vi "Single Tone Microphone Measurements (N Ch).vi"(6 "units settings":T2, 8 "error in":errorcluster, 10 "measurement settings":T4={"Band start"=20.0, "Band stop"=20000.0, "Frequency"=1000.0}, 11 "waveforms":waveform(dbl)[](array[waveform])) -> (0 "error out":errorcluster, 1 "spectra":cluster{"x0":dbl, "dx":dbl, "magnitude":dbl[]}[](array[cluster]), 2 "waveforms":waveform(dbl)[](array[waveform]), 3 "measurements":T1[](array[typedef]))   [LabVIEW 2022 SP3]
uses:
  controls/single tone microphone measurement settings.ctl
  controls/units settings - mic.ctl
  controls/measurement units.ctl
  controls/single tone microphone measurements.ctl
  <vilib>/addons/_NISVFA/_Shared subVIs/Common/SVL Set dB Reference (N Ch - 1 Ref).vi
  <vilib>/addons/_NISVFA/_Spectrum Processing/SVFA Unit Conversion (Complex) (1 Ch).vi
  <vilib>/addons/_NISVFA/_Shared subVIs/Common/SVL Set dB Reference (1 Ch).vi
  <vilib>/addons/_NISVFA/_Shared subVIs/Common/svc_Log View for Spectrum (1Ch).vi
  <vilib>/addons/_NISVFA/_Spectrum Processing/SVFA Unit Conversion (1 Ch).vi
  <vilib>/addons/_NISVFA/_Shared subVIs/Common/svc_Complex Datatype Defaults.vi
  <vilib>/addons/_NISVFA/_Shared subVIs/Common/SVL Set dB Reference (variant).vi
  <vilib>/addons/_NISVFA/_Shared subVIs/Common/svc_Unwrap Phase.vi
  <vilib>/addons/_NISVFA/_Shared subVIs/Common/svc_Convert Spectrum Array to dB.vi
  <vilib>/addons/_NISVFA/_Shared subVIs/Common/svc_Spectrum Units.vi
  <vilib>/addons/_NISVFA/_Spectrum Processing/subVIs/svfa_Conversion Utility (spectrum info).vi
  <vilib>/addons/_NISVFA/_Shared subVIs/Common/svc_Format Value (DBL).vi
  <vilib>/addons/_NISVFA/_Shared subVIs/Common/svc_Get Weighting Enum and Labels.vi
  <vilib>/addons/_NISVFA/_Shared subVIs/Common/svc_Engineering Units to Unit Label.vi
  <vilib>/addons/_NISVFA/_Shared subVIs/Common/svc_Surround NonAlpha String with Parentheses.vi
  <vilib>/dlg_ctls.llb/Space Constant.vi
  <vilib>/addons/_NISVFA/_Spectrum Processing/subVIs/svfa_Peak to RMS to Peak2Peak.vi
  <vilib>/addons/_NISVFA/_Spectrum Processing/subVIs/svfa_Mag to Mag2.vi
  <vilib>/addons/_NISVFA/_Spectrum Processing/subVIs/svfa_Linear to dB.vi
  <vilib>/addons/_NISVFA/_Spectrum Processing/subVIs/svfa_dBrefA to dBrefB.vi
  <vilib>/addons/_NISVFA/_Spectrum Processing/subVIs/svfa_Spectrum to Spectral Density.vi
  <vilib>/addons/_NISVFA/_Shared subVIs/Common/svc_Unit Label Lexical Class.vi
  <vilib>/addons/_NISVFA/_Shared subVIs/Common/svc_Window Parameters.vi
  <vilib>/addons/_NISVFA/_Shared subVIs/Common/svc_Caller VI Returned in Error Source.vi
  <vilib>/addons/Sound and Vibration/svt_Level/SVL Leq Sound Level (1 Ch).vi
  <vilib>/addons/Sound and Vibration/svt_Distortion/SVT SNR without Harmonics (Time) (1 Ch).vi
  <vilib>/addons/_NISVFA/_Spectrum Processing/SVFA Extract Single Tone Information (Complex) (1 Ch).vi
  <vilib>/Analysis/4window.llb/window parameters.vi
  <vilib>/Analysis/4window.llb/Window Properties.vi
  <vilib>/Analysis/4window.llb/Window Properties by Name.vi
  <vilib>/addons/Sound and Vibration/svt_Distortion/SoundVib_Distortion.lvlib
  <vilib>/addons/Sound and Vibration/svt_Level/SoundVib_SoundLevel.lvlib
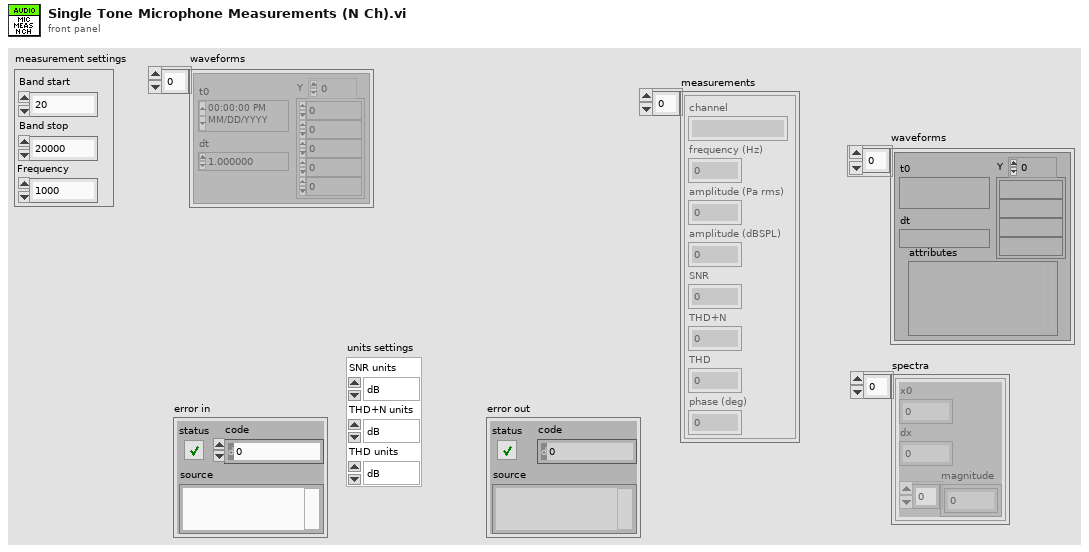
[diagram p1: front panel]
types:
  T1 = typedef "single tone microphone measurements.ctl" = cluster{"channel":string, "frequency (Hz)":dbl, "amplitude (Pa rms)":dbl, "amplitude (dBSPL)":dbl, "SNR":dbl, "THD+N":dbl, "THD":dbl, "phase (deg)":dbl}
  T2 = typedef "units settings - mic.ctl" = cluster{"SNR units":T3, "THD+N units":T3, "THD units":T3}
  T3 = typedef "measurement units.ctl" = enum32{"dB", "x/y"}
  T4 = typedef "single tone microphone measurement settings.ctl" = cluster{"Band start":dbl, "Band stop":dbl, "Frequency":dbl}
  T5 = cluster{"start frequency":dbl, "stop frequency":dbl}
  T6 = cluster{"SNR units":enum16{"dB", "linear ratio", "%"}, "detected fundamental amplitude units":enum16{"EU rms", "EU peak", "EU peak-peak"}}
  T7 = enum16{"no change", "spectrum", "spectral density"}
  T8 = cluster{"linear/dB":enum16{"no change", "linear", "dB"}, "dB reference (0: no change)":dbl, "power/magnitude":enum16{"no change", "power", "magnitude"}, "view":enum16{"no change", "rms", "peak", "peak-peak"}}
  T9 = typedef "svc_Spectrum Info.ctl" = cluster{"channel name":string, "description":string, "x-axis units":T10, "spectral info":cluster{"spectrum type":T11, "linear/dB":enum16{"linear", "dB"}, "window":u16, "window size":i32, "FFT size":i32}, "engineering units":T12, "custom label":string, "dB reference [EU]":dbl, "peak units":enum16{"rms", "peak", "peak-peak"}, "weighting filter":T13, "spectral density?":bool, "unit label":string, "spectrum skewed?":bool, "complimentary spectrum units":T14}
  T10 = typedef "svc_X-Axis Units.ctl" = u16
  T11 = typedef "svc_Spectrum Type.ctl" = enum16{"FFT Spectrum [complex]", "Amplitude [Magnitude]", "Power [Magnitude^2]", "Cross Spectrum [complex]", "Frequency Response [Complex]"}
  T12 = typedef "svc_Engineering Units Text Ring.ctl" = u16
  T13 = typedef "svc_Weighting Filter Text Ring.ctl" = u16
  T14 = typedef "svc_Complimentary Spectrum Units.ctl" = enum16{"none", "radians", "degrees", "cycles", "imaginary"}
  T15 = cluster{"complex spectrum response":cluster{"f0":dbl, "df":dbl, "complex spectrum":cdb[]}, "spectrum info":T9}
  T16 = cluster{"frequency [Hz]":dbl, "amplitude [EU pk]":dbl, "phase (deg)":dbl}
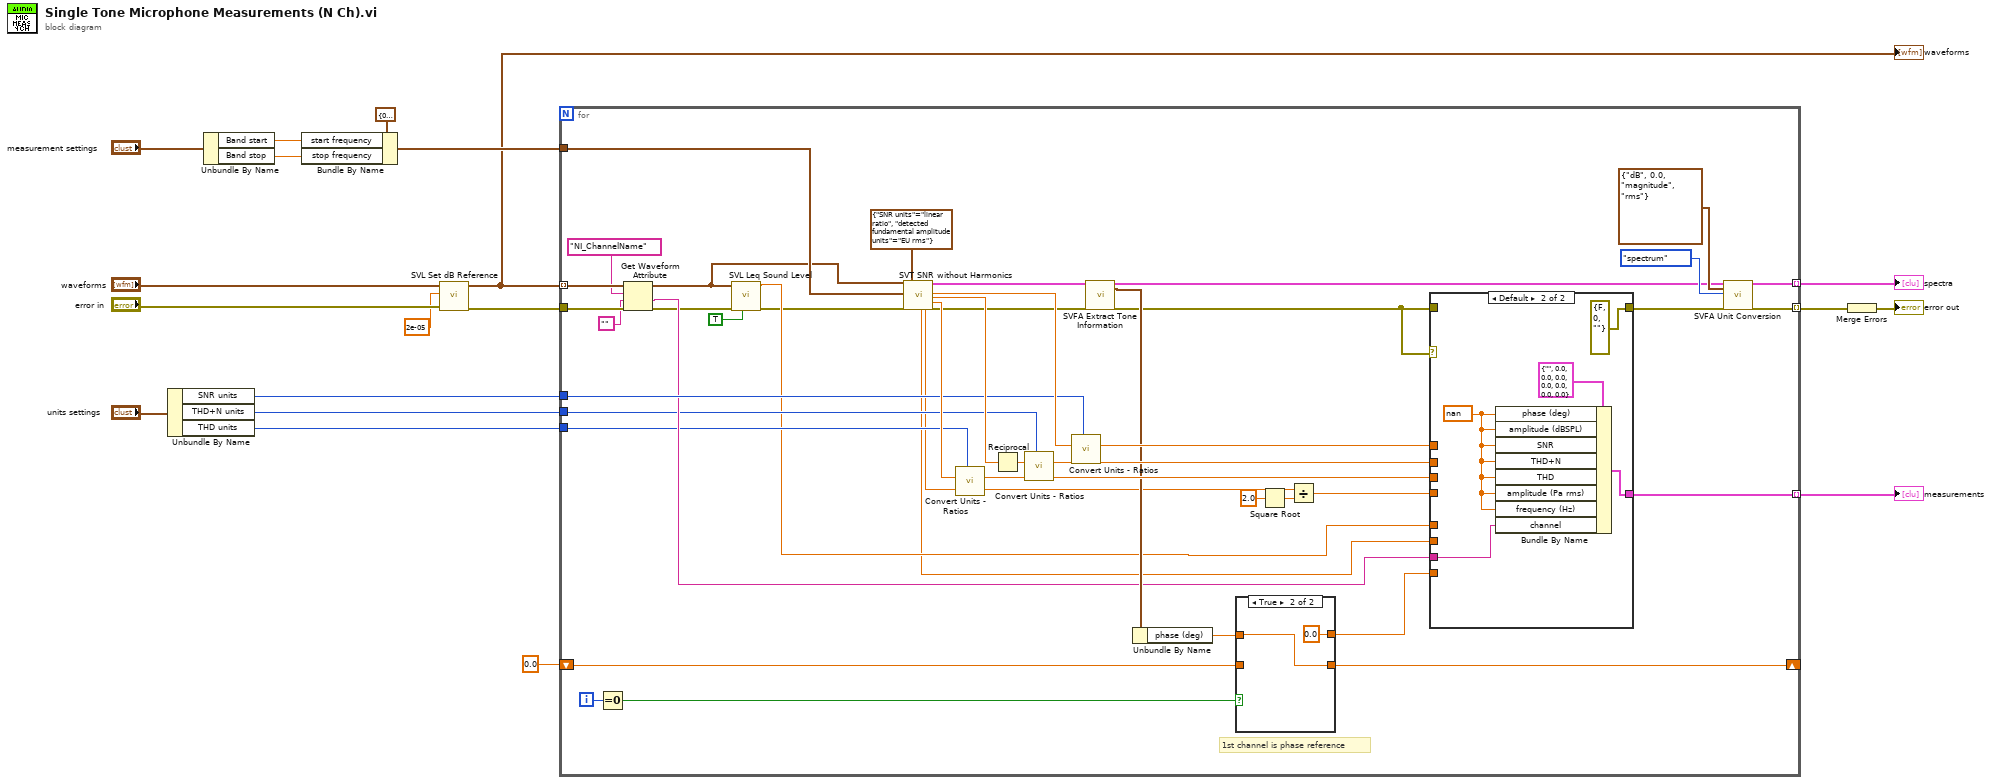
[diagram p0: block diagram]
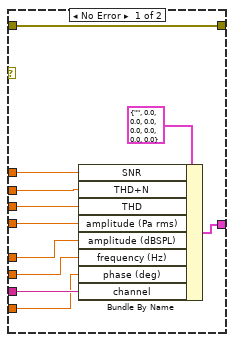
[diagram p2: hidden frame]
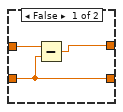
[diagram p3: hidden frame]
diagram:
  n1 = Unbundle By Name("units settings") -> ("SNR units"=w3:T3, "THD+N units"=w11:T3, "THD units"=w10:T3)
  n2 = Unbundle By Name("measurement settings") -> ("Band start"=w18:dbl, "Band stop"=w19:dbl)
  n3 = Bundle By Name(cluster=T5 {"start frequency"=0.0, "stop frequency"=0.0} ("frequency range"), "start frequency"=w18, "stop frequency"=w19) -> (w16:T5)
  n4 = call-poly <vilib>:"SVL Set dB Reference.vi"("error in (no error)"="error in", "dB reference [EU]"=2e-05, "scaled signals in [EU]"="waveforms") -> ("error out"=w14:errorcluster, "scaled signals out [EU]"=w8:waveform(dbl)[])  [unwired: 7 in]
  "waveforms" <- w8
  n5 = for {
    tunnel: w16 -> [w60]
    tunnel: [w59] -> w1 mode=indexing
    tunnel: w11 -> [w30]
    tunnel: w10 -> [w31]
    tunnel: w3 -> [w51]
    tunnel: [w32] -> w6 mode=indexing
    tunnel: w8 -> [w39] mode=indexing
    shift-right: [w41] -> _
    shift-left: 0.0 -> [w43]
    tunnel: w14 -> [w38]
    tunnel: [w33] -> w4 mode=indexing
    i -> [w45]
    # "1st channel is phase reference"
    n6 = Equal To 0?(x=w45) -> (x = 0?=w44:bool)
    n7 = Get Waveform Attribute(4:w38, 5:"", 6:"NI_ChannelName" ("name"), 7:w39) -> (0:w28:errorcluster, 1:w35:string, 3:w20:waveform(dbl))  [unwired: 1 out]
    n8 = call-poly <vilib>:"SVL Leq Sound Level.vi"("restart averaging (F)"=TRUE, "error in (no error)"=w28, "scaled signal [EU]"=w20) -> ("error out"=w21:errorcluster, "Leq sound level [dB EU]"=w26:dbl)  [unwired: 6 in, 1 out]
    n9 = call-poly <vilib>:"SVT SNR without Harmonics.vi"("scaled signal [EU]"=w20, "frequency range"=w60, "error in (no error)"=w21, "desired units"=T6 {"SNR units"=enum."linear ratio", "detected fundamental amplitude units"=enum."EU rms"}) -> ("detected fundamental\nfrequency [Hz]"=w23:dbl, "detected fundamental\namplitude"=w22:dbl, "complex spectrum"=w29:T15, "SNR (without harmonics)"=w58:dbl, "SINAD"=w55:dbl, "THD"=w53:dbl, "error out"=w47:errorcluster)  [unwired: 8 in, 1 out]
    n10 = call "Convert Units - Ratios.vi"("gain units"=w31, "linear ratio"=w53) -> ("converted ratio"=w52:dbl)  [unwired: 9 in]
    n11 = Reciprocal(x=w55) -> (1/x=w56:dbl)
    n12 = call "Convert Units - Ratios.vi"("gain units"=w30, "linear ratio"=w56) -> ("converted ratio"=w54:dbl)  [unwired: 9 in]
    n13 = call "Convert Units - Ratios.vi"("gain units"=w51, "linear ratio"=w58) -> ("converted ratio"=w57:dbl)  [unwired: 9 in]
    n14 = call-poly <vilib>:"SVFA Extract Tone Information.vi"("complex spectrum"=w29, "error in"=w47) -> ("complex spectrum"=w25:T15, "detected tone"=w46:T16, "error out"=w24:errorcluster)  [unwired: 14 in, 1 out]
    n15 = Unbundle By Name(w46) -> ("phase (deg)"=w42:dbl)
    n16 = case shown="True" w44 {
      tunnel: w43 -> [w81 _]
      tunnel: w42 -> [w82 w84]
      tunnel: [w80 0.0] -> w40
      tunnel: [w81 w84] -> w41
      frame False {
        n17 = Subtract(x=w82, y=w81) -> (x-y=w80:dbl)
      }
      frame True {
      }
    }
    n18 = Square Root(x=2.0 ("y")) -> (sqrt(x)=w50:dbl)
    n19 = Divide(x=w22, y=w50) -> (x/y=w48:dbl)
    n20 = case shown="Default" w24 {
      tunnel: [w73 w78] -> w59
      tunnel: w57 -> [w72 _]
      tunnel: w54 -> [w71 _]
      tunnel: w52 -> [w70 _]
      tunnel: w23 -> [w67 _]
      tunnel: w48 -> [w69 _]
      tunnel: w40 -> [w65 _]
      tunnel: w35 -> [w66 w77]
      tunnel: w24 -> [w68 _]
      tunnel: [w68 errorcluster {"status"=FALSE, "code"=0, "source"=""} ("error out")] -> w34
      tunnel: w26 -> [w64 _]
      frame No Error {
        n21 = Bundle By Name(cluster=T1 {"channel"="", "frequency (Hz)"=0.0, "amplitude (Pa rms)"=0.0, "amplitude (dBSPL)"=0.0, "SNR"=0.0, "THD+N"=0.0, "THD"=0.0, "phase (deg)"=0.0} ("results"), "SNR"=w72, "THD+N"=w71, "THD"=w70, "amplitude (Pa rms)"=w69, "amplitude (dBSPL)"=w64, "frequency (Hz)"=w67, "phase (deg)"=w65, "channel"=w66) -> (w73:T1)
      }
      frame Default {
        w75 = nan ("SFDR (dBc)")
        n22 = Bundle By Name(cluster=T1 {"channel"="", "frequency (Hz)"=0.0, "amplitude (Pa rms)"=0.0, "amplitude (dBSPL)"=0.0, "SNR"=0.0, "THD+N"=0.0, "THD"=0.0, "phase (deg)"=0.0} ("results"), "phase (deg)"=w75, "amplitude (dBSPL)"=w75, "SNR"=w75, "THD+N"=w75, "THD"=w75, "amplitude (Pa rms)"=w75, "frequency (Hz)"=w75, "channel"=w77) -> (w78:T1)
      }
    }
    n23 = call-poly <vilib>:"SVFA Unit Conversion.vi"("complex spectrum"=w25, "desired scaling"=T8 {"linear/dB"=enum."dB", "dB reference (0: no change)"=0.0, "power/magnitude"=enum."magnitude", "view"=enum."rms"}, "spectral density desired"=T7."spectrum", "error in (no error)"=w34) -> ("converted spectrum"=w32:cluster{"x0":dbl, "dx":dbl, "magnitude":dbl[]}, "error out"=w33:errorcluster)  [unwired: 10 in, 4 out]
  }
  "spectra" <- w6
  "measurements" <- w1
  n24 = Merge Errors(w4) -> (→"error out":errorcluster)
